vi "cleanSpecificError.vi"(4 "error out":errorcluster, 5 "error code":i32=56) -> (0 "error":bool, 1 "error IO":errorcluster)   [LabVIEW 2011]
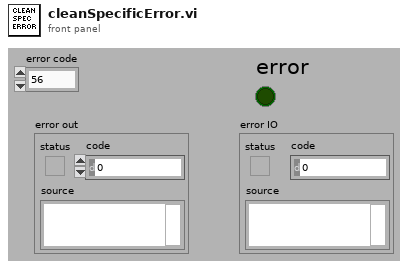
[diagram p1: front panel]
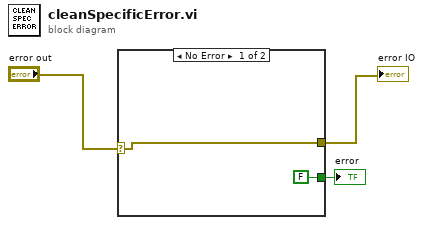
[diagram p0: block diagram]
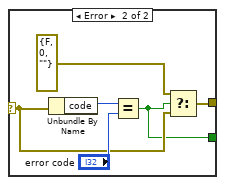
[diagram p2: hidden frame]
diagram:
  n1 = case shown="No Error" "error out" {
    selector: "error out" -> [w5 w8]
    tunnel: [w5 w7] -> w3
    tunnel: [FALSE w6] -> w1
    frame No Error {
    }
    frame Error {
      n2 = Unbundle By Name(w8) -> ("code"=w11:i32)
      n3 = Equal?(x=w11, y="error code") -> (x = y?=w6:bool)
      n4 = Select(t=errorcluster {"status"=FALSE, "code"=0, "source"=""} ("error IO"), s=w6, f=w8) -> (s? t:f=w7:errorcluster)
    }
  }
  "error IO" <- w3
  "error" <- w1
